vi "Alarms.GetList.vi"(10 "Target":string, 11 "GatewayIP Address":string) -> (0 "error out":errorcluster, 3 "AlarmList":string[](array[string]))   [LabVIEW 2013, in "MiscHelperVIs.lvlib"]
uses:
  MiscHelperVIs.lvlib
  <vilib>/NI Veristand/Execution/AlarmManager/NI_VS AlarmManager ExecutionAPI.lvlib
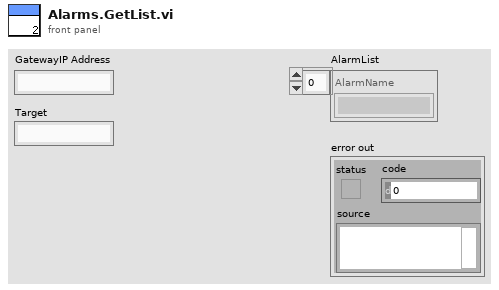
[diagram p1: front panel]
types:
  T1 = typedef "NI_VS AlarmManager ExecutionAPI.lvlib/AlarmManagerAPI.ctl" = refnum<k24>
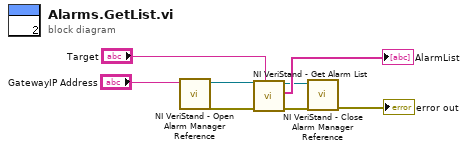
[diagram p0: block diagram]
diagram:
  n1 = call <vilib>:"NI VeriStand - Open Alarm Manager Reference.vi"("Gateway IP Address (\"\": localhost)"="GatewayIP Address") -> ("error out"=w7:errorcluster, "AlarmManager"=w6:T1)  [unwired: 9 in]
  n2 = call <vilib>:"NI VeriStand - Get Alarm List.vi"("Target"="Target", "error in (no error)"=w7, "AlarmManager in"=w6) -> ("error out"=w2:errorcluster, "alarms"=→"AlarmList":string[], "AlarmManager out"=w3:T1)  [unwired: 6 in]
  n3 = call <vilib>:"NI VeriStand - Close Alarm Manager Reference.vi"("error in (no error)"=w2, "AlarmManager"=w3) -> ("error out"=→"error out":errorcluster)  [unwired: 9 in]
